vi "FPGA_DIOTest.vi"() -> ()   [LabVIEW 2014]
uses:
  <vilib>/rvi/Emulation/niFpgaGetClockAttributes.vi
  <vilib>/rvi/Emulation/niFpgaSctlEmulationGetInTimedLoop.vi
  <vilib>/rvi/Emulation/niFpgaEmulationReportErrorSimple.vi
  <vilib>/rvi/eio/common/nirviEmuTemplateMethod_errors.vi
  <vilib>/rvi/Emulation/niFpgaCriticalErrorInLSC.vi
  <vilib>/eio/EIONode/EIONode.xnode
panel:
  out "Boolean":bool
  in  "Count(mSec)":u32=1000
  in  "stop":bool
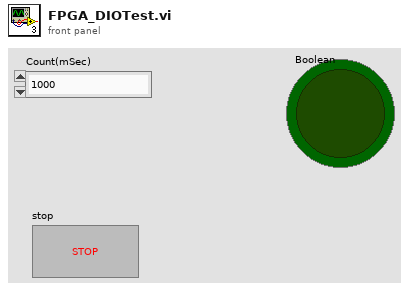
[diagram p1: front panel]
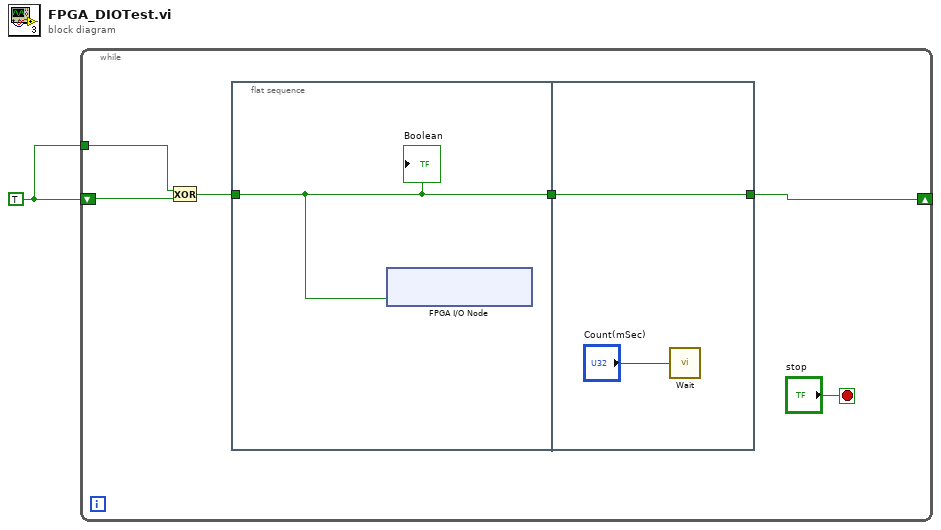
[diagram p0: block diagram]
diagram:
  w1 = TRUE
  n1 = while {
    tunnel: w1 -> [w5]
    shift-right: [w2] -> _
    shift-left: w1 -> [w6]
    stop <- "stop" stop-if-true
    n2 = Exclusive Or(1:w6, 2:w5) -> (0:w4:bool)
    n3 = flat-sequence {
      tunnel: w4 -> [w8]
      tunnel: [w8] -> w3
      tunnel: w3 -> [w9]
      tunnel: [w9] -> w2
      frame #0 {
        n4 = xnode "FPGA I/O Node"("Connector0/DIO0"=w8) -> ()  [unwired: 1 in, 1 out]
        "Boolean" <- w8
      }
      frame #1 {
        n5 = call "Wait"("Count(mSec)"="Count(mSec)") -> ()  [unwired: 1 out]
      }
    }
  }
